vi "Limits Page.vi"(8 "error in (no error)":errorcluster, 10 "LBCB Number":T2) -> (0 "error out":errorcluster)   [LabVIEW 2009]
uses:
  lib/Limits/Faults List Actions.ctl
  lib/Limits/Lower Upper Select.ctl
  lib/Limits/Slider Messages.ctl
  lib/Limits/Limit Slider.ctl
  lib/Data Access Objects/Metadata/LBCB Number.ctl
  lib/Data Access Objects/Limits/DofTypes.ctl
panel:
  out "Messages":string
  in  "Ok":bool
  in  "DofType":T1
  in  "Limit Slider 6":T3 {"Slide" scale=-900.0..900.0 scale format="%#_6f"}
  in  "Limit Slider 5":T3 {"Slide" scale=-900.0..900.0 scale format="%#_6f"}
  in  "Limit Slider 4":T3 {"Slide" scale=-900.0..900.0 scale format="%#_6f"}
  in  "Limit Slider 3":T3 {"Slide" scale=-900.0..900.0 scale format="%#_6f"}
  in  "Limit Slider 2":T3 {"Slide" scale=-900.0..900.0 scale format="%#_6f"}
  in  "Limit Slider 1":T3 {"Slide" scale=-900.0..900.0 scale format="%#_6f"}
  # "Lower"
  # "Higher"
  # "Current"
  # "Global"
  # "Local"
  # "Lower"
  # "Higher"
  # "Current"
  # "Global"
  # "Local"
  # "Lower"
  # "Higher"
  # "Current"
  # "Global"
  # "Local"
  # "Lower"
  # "Higher"
  # "Current"
  # "Global"
  # "Local"
  # "Lower"
  # "Higher"
  # "Current"
  # "Global"
  # "Local"
  # "Lower"
  # "Higher"
  # "Current"
  # "Global"
  # "Local"
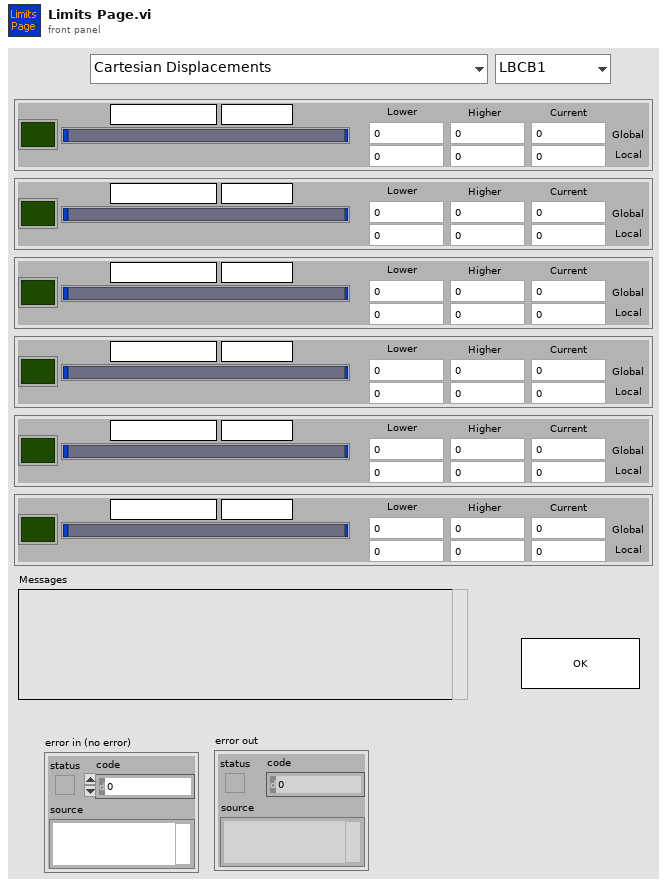
[diagram p1: front panel]
types:
  T1 = typedef "DofTypes.ctl" = enum16{"Cartesian Displacements", "Cartesian Forces & Moments", "Actuator Displacements", "Actuator Forces"}
  T2 = typedef "LBCB Number.ctl" = enum16{"LBCB1", "LBCB2"}
  T3 = typedef "Limit Slider.ctl" = cluster{"Slide":cluster{dbl, dbl, dbl, dbl}, "Global Lo":dbl, "Global Hi":dbl, "Local Lo":dbl, "Local Hi":dbl, "Fault":bool, "DofLabel":string, "Units":string, "Global Actual":dbl, "Local Actual":dbl}
  T4 = typedef "Slider Messages.ctl" = enum16{"Update Display", "Exit", "Nothing"}
  T5 = typedef "Faults List Actions.ctl" = enum16{"Init", "Add", "Remove", "Get List"}
  T6 = typedef "Fault Id.ctl" = cluster{"Fault Type":T7, "LBCB Number":T2, "Index":u32, "Space Type":T8}
  T7 = typedef "Fault Type.ctl" = enum16{"None", "Command", "Displacement", "Force"}
  T8 = typedef "Space Type.ctl" = enum16{"Actuator", "Cartesian"}
  T9 = cluster{"[0]":dbl, "[1]":dbl, "[2]":dbl, "[3]":dbl, "[4]":dbl, "[5]":dbl, "[6]":dbl, "[7]":dbl, "[8]":dbl}[]
  T10 = cluster{"[0]":dbl, "[1]":dbl, "[2]":dbl, "[3]":dbl}
  T11 = typedef "Lower Upper Select.ctl" = enum16{"Lower", "Upper"}
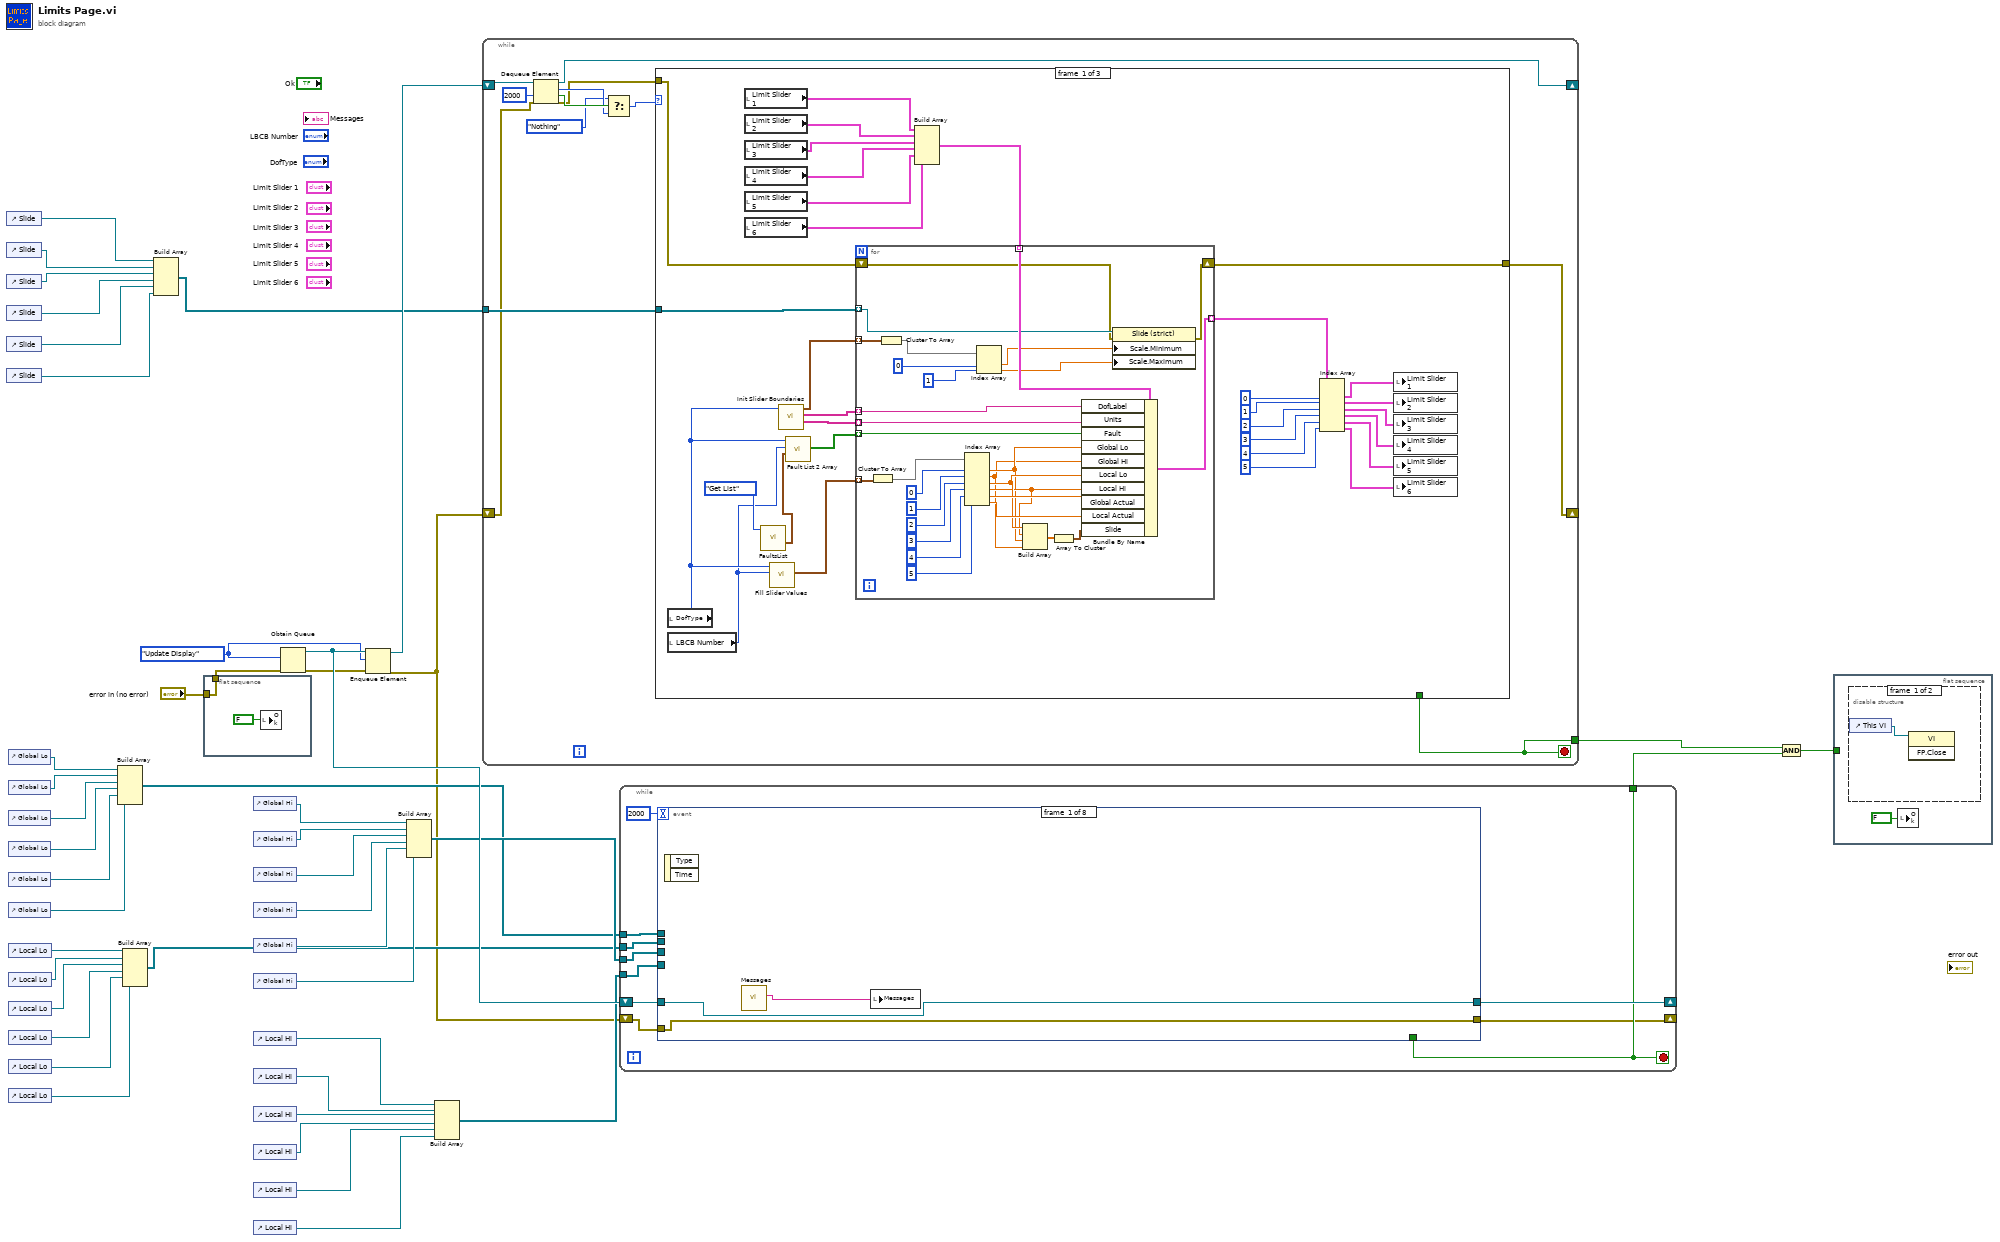
[diagram p0: block diagram]
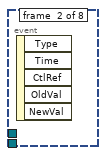
[diagram p3: hidden frame]
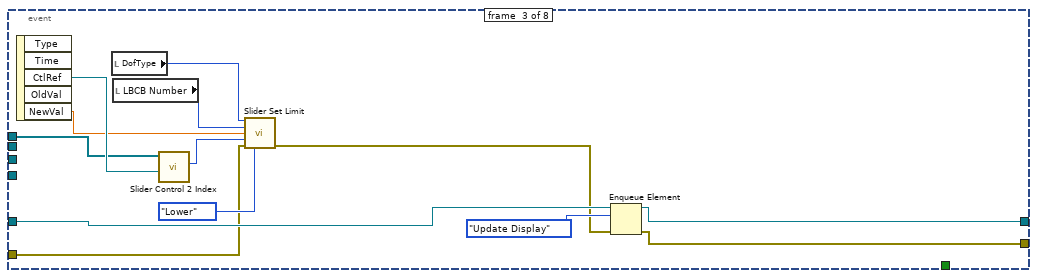
[diagram p4: hidden frame]
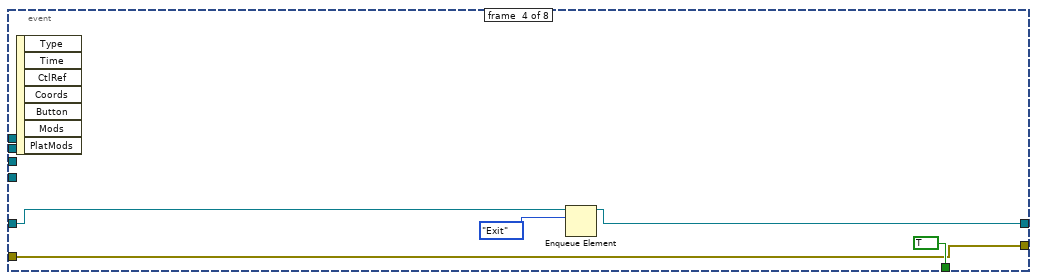
[diagram p5: hidden frame]
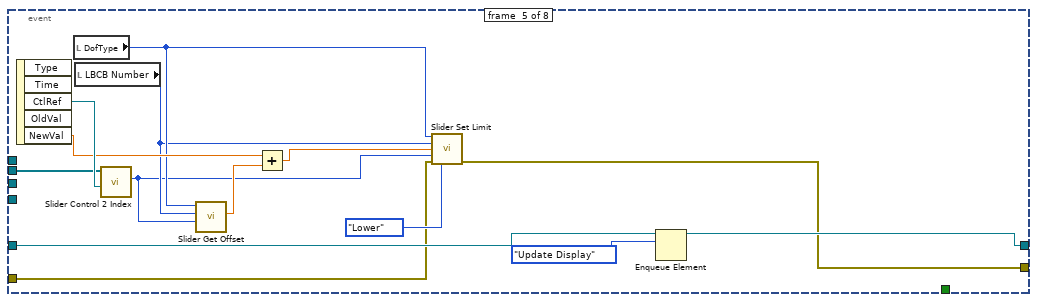
[diagram p6: hidden frame]
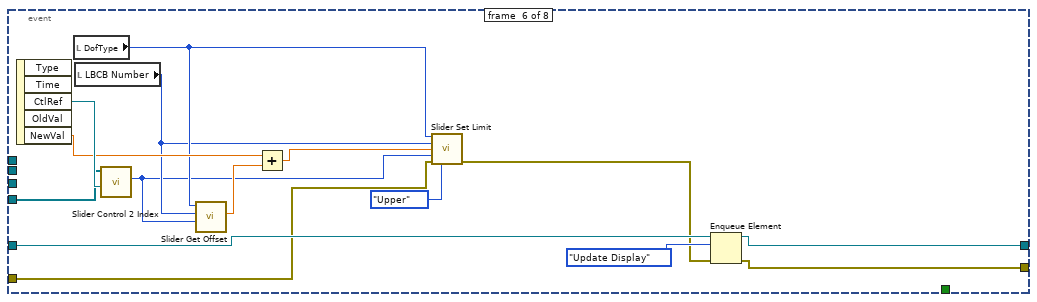
[diagram p7: hidden frame]
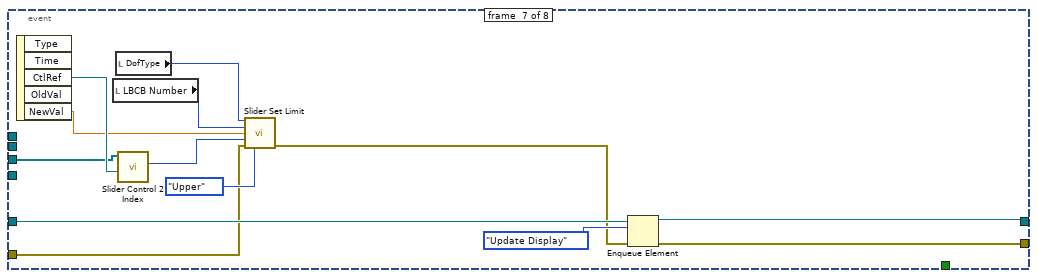
[diagram p8: hidden frame]
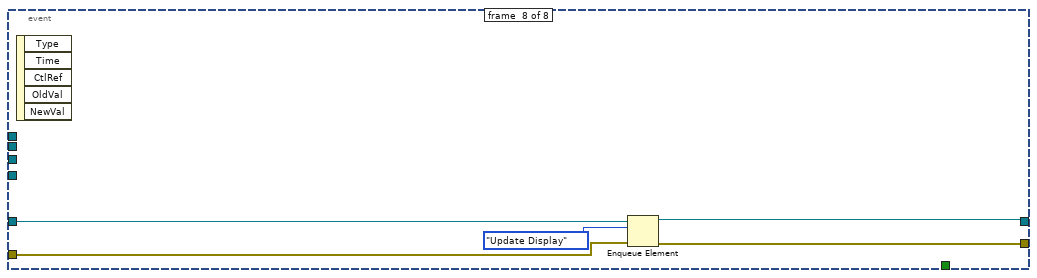
[diagram p9: hidden frame]
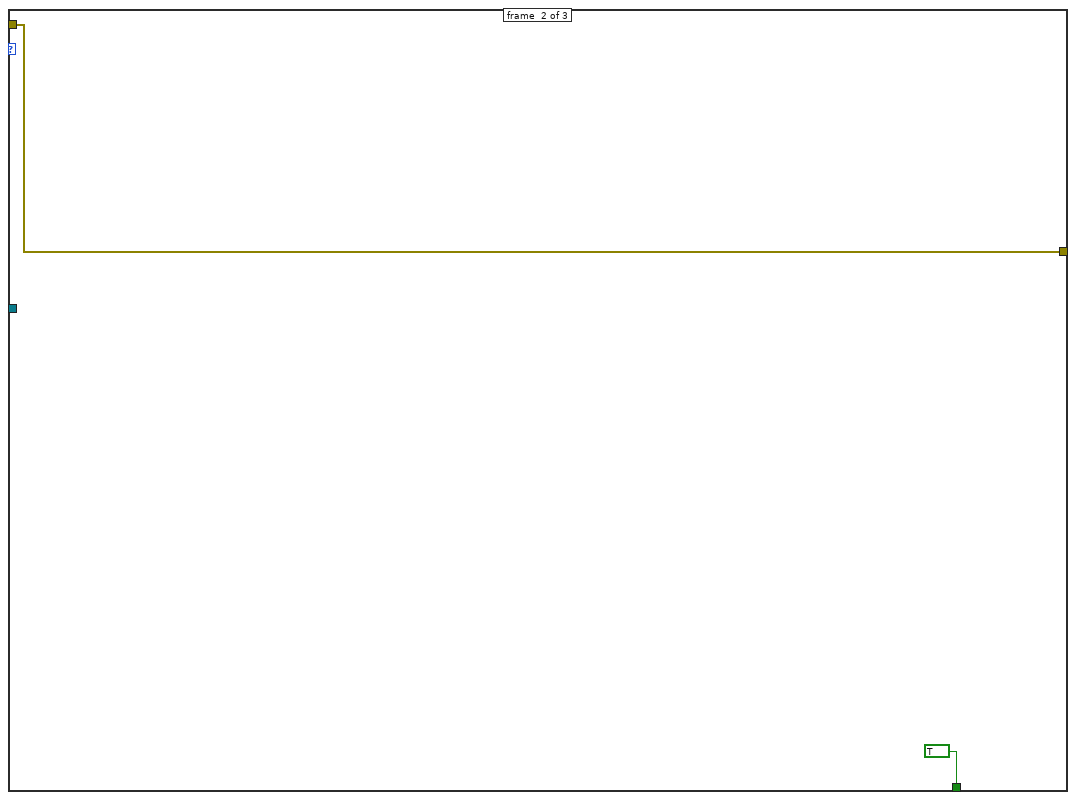
[diagram p10: hidden frame]
diagram:
  w40 = Slider_Messages."Update Display" ("Slider Message")
  n1 = control-ref of="Slide"() -> (w39:refnum<vi>)
  n2 = control-ref of="Slide"() -> (w38:refnum<vi>)
  n3 = control-ref of="Slide"() -> (w37:refnum<vi>)
  n4 = control-ref of="Slide"() -> (w36:refnum<vi>)
  n5 = control-ref of="Slide"() -> (w35:refnum<vi>)
  n6 = control-ref of="Slide"() -> (w34:refnum<vi>)
  n7 = control-ref of="Global Lo"() -> (w32:refnum<vi>)
  n8 = control-ref of="Global Lo"() -> (w31:refnum<vi>)
  n9 = control-ref of="Global Lo"() -> (w30:refnum<vi>)
  n10 = control-ref of="Global Lo"() -> (w29:refnum<vi>)
  n11 = control-ref of="Global Lo"() -> (w28:refnum<vi>)
  n12 = control-ref of="Global Lo"() -> (w27:refnum<vi>)
  n13 = control-ref of="Local Lo"() -> (w26:refnum<vi>)
  n14 = control-ref of="Local Lo"() -> (w25:refnum<vi>)
  n15 = control-ref of="Local Lo"() -> (w24:refnum<vi>)
  n16 = control-ref of="Local Lo"() -> (w23:refnum<vi>)
  n17 = control-ref of="Local Lo"() -> (w22:refnum<vi>)
  n18 = control-ref of="Local Lo"() -> (w21:refnum<vi>)
  n19 = Build Array(w32, w31, w30, w29, w28, w27) -> (w5:refnum<vi>[])
  n20 = Build Array(w26, w25, w24, w23, w22, w21) -> (w6:refnum<vi>[])
  n21 = Build Array(w39, w38, w37, w36, w35, w34) -> (w33:refnum<vi>[])
  n22 = flat-sequence {
    tunnel: "error in (no error)" -> [w47]
    tunnel: [w47] -> w3
    frame #0 {
      n23 = local write "Ok"(FALSE ("Ok")) -> ()
    }
  }
  n24 = control-ref of="Global Hi"() -> (w20:refnum<vi>)
  n25 = control-ref of="Global Hi"() -> (w19:refnum<vi>)
  n26 = control-ref of="Global Hi"() -> (w18:refnum<vi>)
  n27 = control-ref of="Global Hi"() -> (w17:refnum<vi>)
  n28 = control-ref of="Global Hi"() -> (w16:refnum<vi>)
  n29 = control-ref of="Global Hi"() -> (w15:refnum<vi>)
  n30 = control-ref of="Local Hi"() -> (w14:refnum<vi>)
  n31 = control-ref of="Local Hi"() -> (w13:refnum<vi>)
  n32 = control-ref of="Local Hi"() -> (w12:refnum<vi>)
  n33 = control-ref of="Local Hi"() -> (w11:refnum<vi>)
  n34 = control-ref of="Local Hi"() -> (w10:refnum<vi>)
  n35 = control-ref of="Local Hi"() -> (w9:refnum<vi>)
  n36 = Obtain Queue(element data type=w40, error in (no error)=w3) -> (queue out=w45:refnum<queue>, error out=w2:errorcluster)  [unwired: 3 in, 1 out]
  n37 = Enqueue Element(queue=w45, element=w40, error in (no error)=w2) -> (queue out=w41:refnum<queue>, error out=w1:errorcluster)  [unwired: 1 in, 1 out]
  n38 = Build Array(w20, w19, w18, w17, w16, w15) -> (w7:refnum<vi>[])
  n39 = Build Array(w14, w13, w12, w11, w10, w9) -> (w8:refnum<vi>[])
  n40 = while {
    tunnel: w33 -> [w59]
    shift-right: [w56] -> _
    shift-left: w41 -> [w58]
    tunnel: [w51] -> w44
    shift-right: [w48] -> _
    shift-left: w1 -> [w50]
    stop <- w51 stop-if-true
    n41 = Dequeue Element(queue=w58, timeout in ms (-1)=2000, error in (no error)=w50) -> (queue out=w56:refnum<queue>, element=w54:T4, timed out?=w55:bool, error out=w49:errorcluster)
    n42 = Select(t=Slider_Messages."Nothing", s=w55, f=w54) -> (s? t:f=w52:T4)
    n43 = case shown="\"Exit\"" w52 {
      tunnel: w59 -> [w90 _ _]
      tunnel: [_ TRUE _] -> w51
      tunnel: w49 -> [w61 w122 w124]
      tunnel: [w60 w122 w124] -> w48
      frame #0 {
        n44 = local read "DofType"() -> (w64:T1)
        n45 = local read "LBCB Number"() -> (w63:T2)
        n46 = local read "Limit Slider 1"() -> (w76:T3)
        n47 = local read "Limit Slider 2"() -> (w75:T3)
        n48 = local read "Limit Slider 3"() -> (w74:T3)
        n49 = local read "Limit Slider 4"() -> (w73:T3)
        n50 = local read "Limit Slider 5"() -> (w72:T3)
        n51 = local read "Limit Slider 6"() -> (w71:T3)
        n52 = call "FaultsList.vi"("Limits List Actions"=Faults_List_Actions."Get List") -> ("Fault List"=w65:T6[])  [unwired: 2 in, 8 out]
        n53 = call "Fill Slider Values.vi"("LBCB Number"=w63, "DofType"=w64) -> ("Silder Values"=w62:T9)  [unwired: 9 in]
        n54 = call "Init Slider Boundaries.vi"("DofType"=w64) -> ("Unit Labels"=w68:string[], "Dof Labels"=w69:string[], "Boundaries"=w70:cluster{"[0]":dbl, "[1]":dbl}[])  [unwired: 8 in]
        n55 = call "Fault List 2 Array.vi"("Fault List"=w65, "LBCB Number"=w63, "DofType"=w64) -> ("Faults"=w66:bool[])  [unwired: 8 in]
        n56 = Build Array(w76, w75, w74, w73, w72, w71) -> (w77:T3[])
        n57 = for {
          tunnel: w77 -> [w121] mode=indexing
          tunnel: [w120] -> w91 mode=indexing
          tunnel: w90 -> [w102] mode=indexing
          tunnel: w66 -> [w119] mode=indexing
          tunnel: w70 -> [w118] mode=indexing
          tunnel: w69 -> [w114] mode=indexing
          tunnel: w68 -> [w113] mode=indexing
          tunnel: w62 -> [w112] mode=indexing
          shift-right: [w92] -> w60
          shift-left: w61 -> [w93]
          n58 = Cluster To Array(cluster=w112) -> (array=w111:dbl[])
          n59 = Cluster To Array(cluster=w118) -> (array=w115:dbl[])
          n60 = Index Array(array=w111, index #1=0 ("index"), index #2=1 ("index"), index #3=2 ("index"), index #4=3 ("index"), index #5=4 ("index"), index #6=5 ("index")) -> (element #1=w97:dbl, element #2=w96:dbl, element #3=w99:dbl, element #4=w98:dbl, element #5=w105:dbl, element #6=w103:dbl)
          n61 = Index Array(array=w115, index #1=0 ("index"), index #2=1 ("index")) -> (element #1=w101:dbl, element #2=w100:dbl)
          n62 = Build Array(w99, w98, w97, w96) -> (w95:dbl[])
          n63 = Array To Cluster(array=w95) -> (cluster=w94:T10)
          n64 = Bundle By Name(cluster=w121, "DofLabel"=w114, "Units"=w113, "Fault"=w119, "Global Lo"=w97, "Global Hi"=w96, "Local Lo"=w99, "Local Hi"=w98, "Global Actual"=w105, "Local Actual"=w103, "Slide"=w94) -> (w120:T3)
          n65 = property class="Slide (strict)"(reference=w102, error in=w93, "Scale.Minimum"=w101, "Scale.Maximum"=w100) -> (error out=w92:errorcluster)  [unwired: 1 out]
        }
        n66 = Index Array(array=w91, index #1=0 ("index"), index #2=1 ("index"), index #3=2 ("index"), index #4=3 ("index"), index #5=4 ("index"), index #6=5 ("index")) -> (element #1=w89:T3, element #2=w82:T3, element #3=w81:T3, element #4=w80:T3, element #5=w79:T3, element #6=w78:T3)
        n67 = local write "Limit Slider 1"(w89) -> ()
        n68 = local write "Limit Slider 2"(w82) -> ()
        n69 = local write "Limit Slider 3"(w81) -> ()
        n70 = local write "Limit Slider 4"(w80) -> ()
        n71 = local write "Limit Slider 5"(w79) -> ()
        n72 = local write "Limit Slider 6"(w78) -> ()
      }
      frame #1 {
      }
      frame #2 {
      }
    }
  }
  n73 = while {
    shift-right: [w132] -> _
    shift-left: w45 -> [w133]
    tunnel: [w131] -> w43
    tunnel: w8 -> [w128]
    tunnel: w7 -> [w127]
    tunnel: w6 -> [w129]
    tunnel: w5 -> [w130]
    shift-right: [w125] -> _
    shift-left: w1 -> [w126]
    stop <- w131 stop-if-true
    n74 = event shown="[1] \"Limit Slider 1.Slide\": Value Change" {
      selector: _ -> [_ _ _ _ _ _ _ _]
      dyn-events: _ -> [_ _ _ _ _ _ _ _]
      timeout: 2000 -> [_ _ _ _ _ _ _ _]
      tunnel: w133 -> [w136 _ w143 w154 w160 w176 w190 w201]
      tunnel: [w136 _ w142 w153 w159 w174 w189 w200] -> w132
      tunnel: [_ _ _ TRUE _ _ _ _] -> w131
      tunnel: w130 -> [_ _ w141 _ _ _ _ _]
      tunnel: w129 -> [_ _ _ _ w158 _ _ _]
      tunnel: w128 -> [_ _ _ _ _ w173 _ _]
      tunnel: w127 -> [_ _ _ _ _ _ w188 _]
      tunnel: w126 -> [w135 _ w140 w151 w157 w172 w187 w199]
      tunnel: [w135 _ w138 w151 w156 w170 w185 w198] -> w125
      event #0 {
        n75 = event-data() -> ()  [unwired: 1 in, 2 out]
        n76 = call "Messages.vi"() -> ("Messages"=w137:string)  [unwired: 2 in, 9 out]
        n77 = local write "Messages"(w137) -> ()
      }
      event #1 {
        n78 = event-data() -> ()  [unwired: 1 in, 5 out]
      }
      event #2 {
        n79 = event-data() -> ("CtlRef"=w150:refnum<vi>, "NewVal"=w146:dbl)  [unwired: 1 in, 3 out]
        n80 = local read "DofType"() -> (w147:T1)
        n81 = local read "LBCB Number"() -> (w148:T2)
        n82 = call "Slider Control 2 Index.vi"("Control"=w150, "Controls"=w141) -> ("Index"=w149:i32)  [unwired: 9 in]
        n83 = call "Slider Set Limit.vi"("DofType"=w147, "LBCB Number"=w148, "Value"=w146, "Index"=w149, "error in (no error)"=w140, "Lower/Upper"=Lower_Upper_Select."Lower") -> ("error out"=w139:errorcluster)  [unwired: 9 in]
        n84 = Enqueue Element(queue=w143, element=Slider_Messages."Update Display", error in (no error)=w139) -> (queue out=w142:refnum<queue>, error out=w138:errorcluster)  [unwired: 1 in, 1 out]
      }
      event #3 {
        n85 = event-data() -> ()  [unwired: 1 in, 7 out]
        n86 = Enqueue Element(queue=w154, element=Slider_Messages."Exit") -> (queue out=w153:refnum<queue>)  [unwired: 2 in, 2 out]
      }
      event #4 {
        n87 = event-data() -> ("CtlRef"=w169:refnum<vi>, "NewVal"=w166:dbl)  [unwired: 1 in, 3 out]
        n88 = local read "DofType"() -> (w164:T1)
        n89 = local read "LBCB Number"() -> (w163:T2)
        n90 = call "Slider Control 2 Index.vi"("Control"=w169, "Controls"=w158) -> ("Index"=w162:i32)  [unwired: 9 in]
        n91 = call "Slider Get Offset.vi"("Index"=w162, "LBCB Number"=w163, "DofType"=w164) -> ("Offset"=w165:dbl)  [unwired: 8 in]
        n92 = Add(x=w166, y=w165) -> (x+y=w167:dbl)
        n93 = call "Slider Set Limit.vi"("DofType"=w164, "LBCB Number"=w163, "Value"=w167, "Index"=w162, "error in (no error)"=w157, "Lower/Upper"=Lower_Upper_Select."Lower") -> ("error out"=w156:errorcluster)  [unwired: 9 in]
        n94 = Enqueue Element(queue=w160, element=Slider_Messages."Update Display") -> (queue out=w159:refnum<queue>)  [unwired: 2 in, 2 out]
      }
      event #5 {
        n95 = event-data() -> ("CtlRef"=w184:refnum<vi>, "NewVal"=w181:dbl)  [unwired: 1 in, 3 out]
        n96 = local read "DofType"() -> (w179:T1)
        n97 = local read "LBCB Number"() -> (w178:T2)
        n98 = call "Slider Control 2 Index.vi"("Control"=w184, "Controls"=w173) -> ("Index"=w177:i32)  [unwired: 9 in]
        n99 = call "Slider Get Offset.vi"("Index"=w177, "LBCB Number"=w178, "DofType"=w179) -> ("Offset"=w180:dbl)  [unwired: 8 in]
        n100 = Add(x=w181, y=w180) -> (x+y=w182:dbl)
        n101 = call "Slider Set Limit.vi"("DofType"=w179, "LBCB Number"=w178, "Value"=w182, "Index"=w177, "error in (no error)"=w172, "Lower/Upper"=Lower_Upper_Select."Upper") -> ("error out"=w171:errorcluster)  [unwired: 9 in]
        n102 = Enqueue Element(queue=w176, element=Slider_Messages."Update Display", error in (no error)=w171) -> (queue out=w174:refnum<queue>, error out=w170:errorcluster)  [unwired: 1 in, 1 out]
      }
      event #6 {
        n103 = event-data() -> ("CtlRef"=w197:refnum<vi>, "NewVal"=w193:dbl)  [unwired: 1 in, 3 out]
        n104 = local read "LBCB Number"() -> (w195:T2)
        n105 = local read "DofType"() -> (w194:T1)
        n106 = call "Slider Control 2 Index.vi"("Control"=w197, "Controls"=w188) -> ("Index"=w196:i32)  [unwired: 9 in]
        n107 = call "Slider Set Limit.vi"("DofType"=w194, "LBCB Number"=w195, "Value"=w193, "Index"=w196, "error in (no error)"=w187, "Lower/Upper"=Lower_Upper_Select."Upper") -> ("error out"=w186:errorcluster)  [unwired: 9 in]
        n108 = Enqueue Element(queue=w190, element=Slider_Messages."Update Display", error in (no error)=w186) -> (queue out=w189:refnum<queue>, error out=w185:errorcluster)  [unwired: 1 in, 1 out]
      }
      event #7 {
        n109 = event-data() -> ()  [unwired: 1 in, 5 out]
        n110 = Enqueue Element(queue=w201, element=Slider_Messages."Update Display", error in (no error)=w199) -> (queue out=w200:refnum<queue>, error out=w198:errorcluster)  [unwired: 1 in, 1 out]
      }
    }
  }
  n111 = Compound Arithmetic op=AND(w44, w43) -> (w42:bool)
  n112 = flat-sequence {
    tunnel: w42 -> [_]
    frame #0 {
      n113 = disable-structure shown="Enabled" {
        frame #0 {
          n114 = control-ref of="This VI"() -> (w204:refnum<vi>)
          n115 = invoke class="VI" method="FP.Close"(reference=w204) -> ()  [unwired: 2 in, 3 out]
        }
        frame #1 {
        }
      }
      n116 = local write "Ok"(FALSE ("Ok")) -> ()
    }
  }
